vi "initialise.vi"(8 "error in (no error)":errorcluster, 11 "DL090201FrameScanTrajectory in":refnum<class "TrajectoryDL090201FrameScan.lvclass">) -> (0 "error out":errorcluster, 3 "DL090201FrameScanTrajectory out":refnum<class "TrajectoryDL090201FrameScan.lvclass">)   [LabVIEW 2010, in "TrajectoryDL090201FrameScan.lvclass"]
uses:
  TrajectoryDL090201FrameScan.lvclass
  TrajectoryDL091126GenericVoxel/TrajectoryDL091126GenericVoxel/TrajectoryDL091126GenericVoxel.lvclass
  common/enumerations/x_y_z_enumeration.ctl
  common/enumerations/functional_global_action_enum.ctl
  TrajectoryDL090201FrameScan.lvclass/TrajectoryDL090201FrameScan.ctl
  <vilib>/Analysis/1siggen.llb/Ramp Pattern by Samples.vi
  common/classes/ErrorController/ErrorController/class_data.vi
  common/classes/Box/Box/Box.lvclass
  common/classes/SpaceVector/SpaceVector/SpaceVector.lvclass
  <vilib>/Analysis/NI_AALBase.lvlib
  common/classes/ErrorController/ErrorController/ErrorController.lvclass
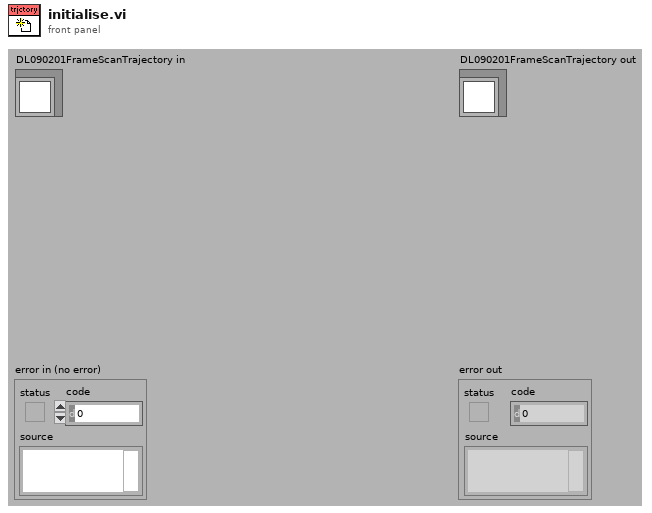
[diagram p1: front panel]
types:
  T1 = typedef "functional_global_action_enum.ctl" = enum16{"get", "set", "reset"}
  T2 = typedef "x_y_z_enumeration.ctl" = enum16{"x", "y", "z"}
  T3 = typedef "space_vector_array.ctl" = dbl[unit][]
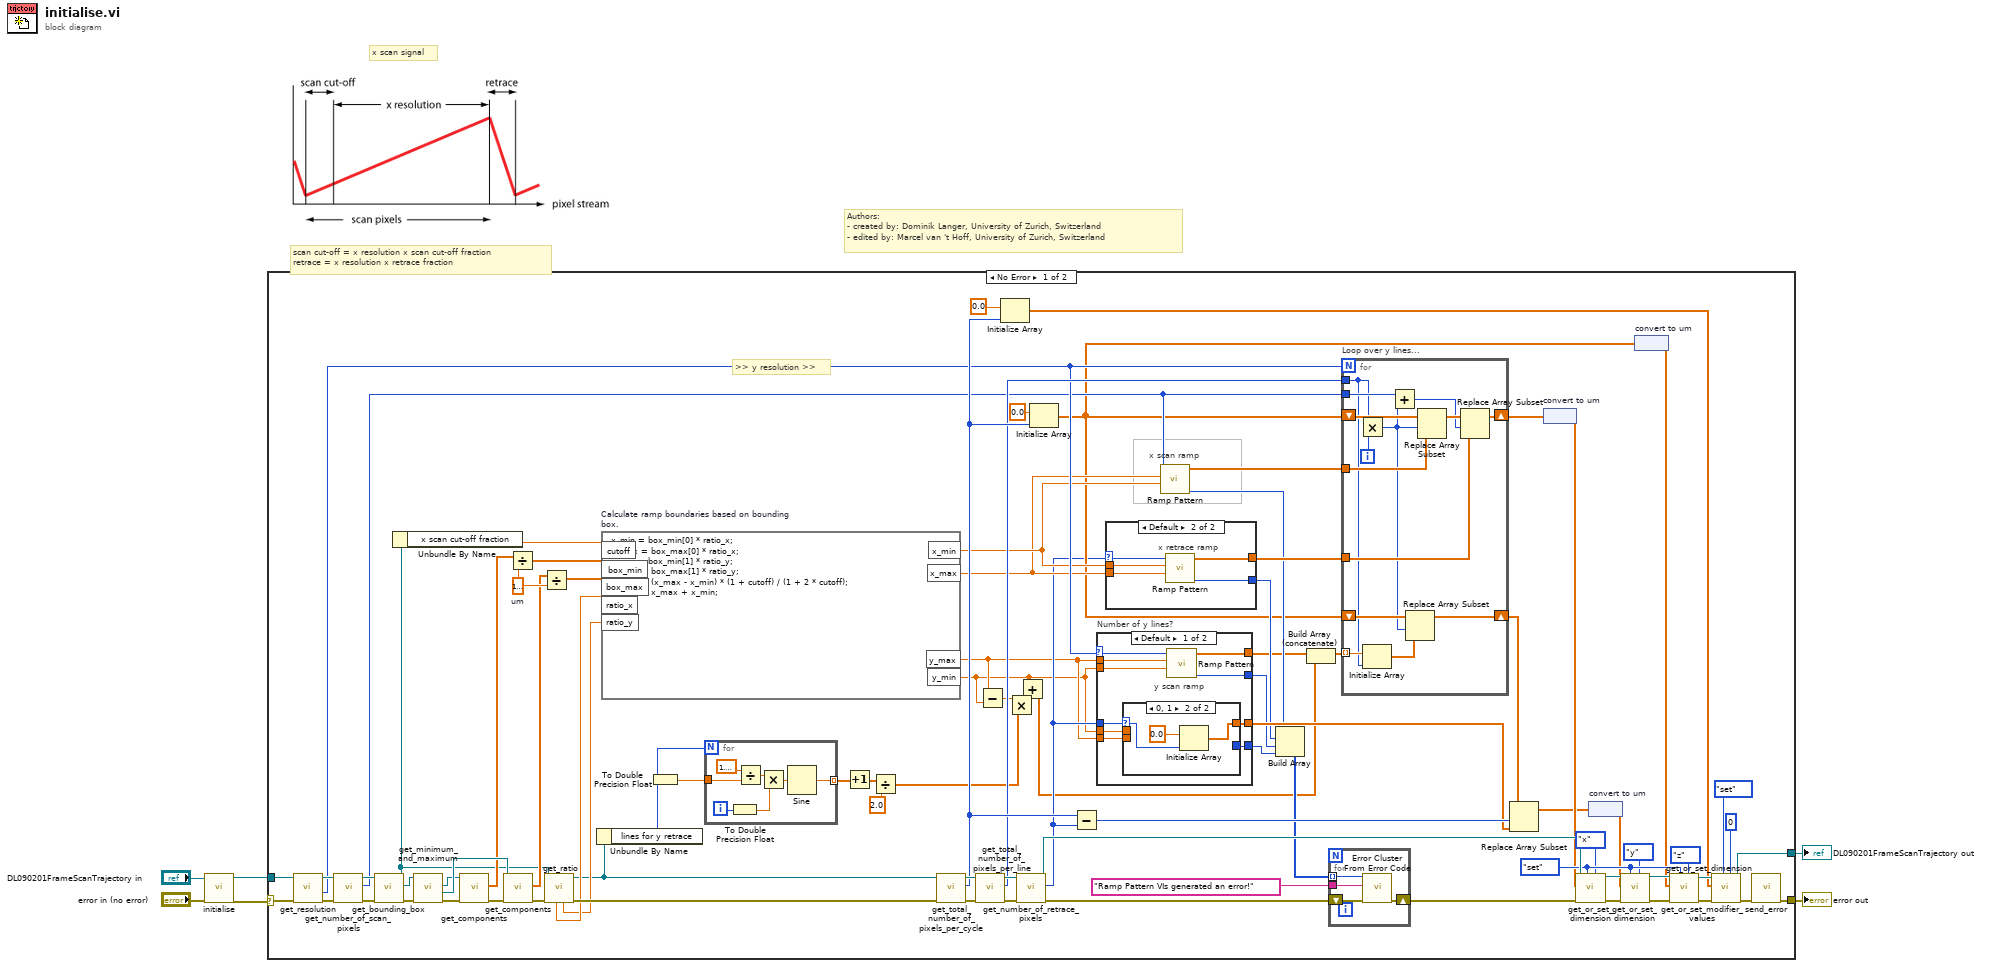
[diagram p0: block diagram]
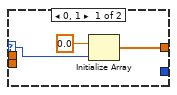
[diagram p2: hidden frame]
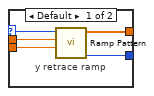
[diagram p3: hidden frame]
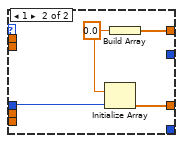
[diagram p4: hidden frame]
diagram:
  # "scan cut-off = x resolution x scan cut-off fraction\nretrace = x resolution x retrace fraction"
  # "x scan signal"
  # "Authors: \n- created by: Dominik Langer, University of Zurich, Switzerland\n- edited by: Marcel van 't Hoff, University of Zurich, Switzerland"
  n1 = call-parent "initialise.vi"("error in (no error)"="error in (no error)", "GenericTrajectory in"="DL090201FrameScanTrajectory in") -> ("error out"=w3:errorcluster, "GenericTrajectory out"=w1:refnum<class "TrajectoryDL090201FrameScan.lvclass">)  [unwired: 8 out]
  n2 = case shown="No Error" w3 {
    selector: w3 -> [w70 w149]
    tunnel: [w46 w149] -> w6
    tunnel: [w48 w148] -> w5
    tunnel: w1 -> [w29 w148]
    frame No Error {
      w61 = functional_global_action_enum."set" ("action")
      w86 = dbl[unit] 1e-06  # um
      # ">> y resolution >>"
      # "x scan ramp"
      n3 = call-dynamic "get_resolution.vi"("error in (no error)"=w70, "TrajectoryDL090201FrameScan in"=w29) -> ("error out"=w69:errorcluster, "y"=w57:i32, "TrajectoryDL090201FrameScan out"=w68:refnum<class "TrajectoryDL090201FrameScan.lvclass">)  [unwired: 7 out]
      n4 = call "get_number_of_scan_pixels.vi"("error in (no error)"=w69, "DL090201FrameScanTrajectory in"=w68) -> ("error out"=w73:errorcluster, "number of scan pixels"=w31:i32, "DL090201FrameScanTrajectory out"=w72:refnum<class "TrajectoryDL090201FrameScan.lvclass">)  [unwired: 7 out]
      n5 = call-dynamic "get_bounding_box.vi"("error in (no error)"=w73, "GenericTrajectory in"=w72) -> ("error out"=w77:errorcluster, "Box.lvclass"=w76:refnum<class "Box.lvclass">, "GenericTrajectory out"=w28:refnum<class "TrajectoryDL090201FrameScan.lvclass">)  [unwired: 7 in]
      n6 = Unbundle By Name(w28) -> ("x scan cut-off fraction"=w30:dbl)
      n7 = call "get_minimum_and_maximum.vi"("error in (no error)"=w77, "Box in"=w76) -> ("error out"=w75:errorcluster, "maximum"=w65:refnum<class "SpaceVector.lvclass">, "minimum"=w64:refnum<class "SpaceVector.lvclass">)  [unwired: 7 out]
      n8 = call "get_components.vi"("error in (no error)"=w75, "SpaceVector in"=w64) -> ("error out"=w74:errorcluster, "x/y/z"=w37:T3)  [unwired: 8 out]
      n9 = call "get_components.vi"("error in (no error)"=w74, "SpaceVector in"=w65) -> ("error out"=w55:errorcluster, "x/y/z"=w33:T3)  [unwired: 8 out]
      n10 = Divide(x=w37, y=w86) -> (x/y=w36:dbl[])
      n11 = Divide(x=w33, y=w86) -> (x/y=w32:dbl[])
      n12 = call-dynamic "get_ratio.vi"("error in (no error)"=w55, "TrajectoryDL090201FrameScan in"=w28) -> ("error out"=w54:errorcluster, "TrajectoryDL090201FrameScan out"=w19:refnum<class "TrajectoryDL090201FrameScan.lvclass">, "y normalised"=w38:dbl, "x normalised"=w39:dbl)  [unwired: 6 out]
      n13 = Unbundle By Name(w19) -> ("lines for y retrace"=w18:i32)
      n14 = formula code="x_min = box_min[0] * ratio_x;\nx_max = box_max[0] * ratio_x;\ny_min = box_min[1] * ratio_y;\ny_max = box_max[1] * ratio_y;\nx_max = (x_max - x_min) * (1 + cutoff) / (1 + 2 * cutoff);\nx_max = x_max + x_min;" "Calculate ramp boundaries based on bounding box."("box_min"=w36, "box_max"=w32, "ratio_x"=w39, "ratio_y"=w38, "cutoff"=w30) -> ("x_min"=w35:dbl, "x_max"=w34:dbl, "y_min"=w11:dbl, "y_max"=w20:dbl)
      n15 = To Double Precision Float(number=w18) -> (double precision float=w17:dbl)
      n16 = for {
        N: w18 -> [_]
        tunnel: [w99] -> w15 mode=indexing
        tunnel: w17 -> [w98]
        i -> [w96]
        n17 = To Double Precision Float(number=w96) -> (double precision float=w95:dbl)
        n18 = Divide(x=1.5707963267948966, y=w98) -> (x/y=w97:dbl)
        n19 = Multiply(x=w97, y=w95) -> (x*y=w94:dbl)
        n20 = Sine(x=w94) -> (sin(x)=w99:dbl)
      }
      n21 = Increment(x=w15) -> (x+1=w14:dbl[])
      n22 = Divide(x=w14, y=2.0) -> (x/y=w10:dbl[])
      n23 = call-dynamic "get_total_number_of_pixels_per_cycle.vi"("error in (no error)"=w54, "TrajectoryDL090201FrameScan in"=w19) -> ("error out"=w81:errorcluster, "total number of pixels per cycle"=w67:i32, "TrajectoryDL090201FrameScan out"=w79:refnum<class "TrajectoryDL090201FrameScan.lvclass">)  [unwired: 7 out]
      n24 = call-dynamic "get_total_number_of_pixels_per_line.vi"("error in (no error)"=w81, "DL090201FrameScanTrajectory in"=w79) -> ("error out"=w80:errorcluster, "total number of pixels per line"=w66:i32, "DL090201FrameScanTrajectory out"=w78:refnum<class "TrajectoryDL090201FrameScan.lvclass">)  [unwired: 7 out]
      n25 = Subtract(x=w20, y=w11) -> (x-y=w16:dbl)
      n26 = Initialize Array(0.0 ("element"), w67) -> (w50:dbl[])
      n27 = Multiply(x=w16, y=w10) -> (x*y=w12:dbl[])
      n28 = call "get_number_of_retrace_pixels.vi"("error in (no error)"=w80, "DL090201FrameScanTrajectory in"=w78) -> ("error out"=w62:errorcluster, "number of retrace pixels"=w21:i32, "DL090201FrameScanTrajectory out"=w63:refnum<class "TrajectoryDL090201FrameScan.lvclass">)  [unwired: 7 out]
      n29 = Add(x=w11, y=w12) -> (x+y=w7:dbl[])
      n30 = Initialize Array(0.0 ("element"), w67) -> (w25:dbl[])
      n31 = Subtract(x=w67, y=w21) -> (x-y=w89:i32)
      n32 = case "Number of y lines?" shown="Default" w57 {
        selector: w57 -> [w113 _]
        tunnel: [w121 w133] -> w8
        tunnel: w20 -> [w120 _]
        tunnel: w11 -> [w119 _]
        tunnel: [w118 _] -> w42
        tunnel: [w117 _] -> w40
        tunnel: [w116 w131] -> w56
        tunnel: w21 -> [w112 w130]
        tunnel: w11 -> [w115 _]
        tunnel: w20 -> [w114 _]
        frame Default {
          # "y scan ramp"
          n33 = case shown="0, 1" w112 {
            selector: w112 -> [w122 w129]
            tunnel: [w126 _] -> w117
            tunnel: [w125 w127] -> w116
            tunnel: w115 -> [w124 _]
            tunnel: w114 -> [w123 _]
            frame Default {
              # "y retrace ramp"
              n34 = call-poly <vilib>:"Ramp Pattern.vi"("start"=w123, "end"=w124, "samples"=w122) -> ("error"=w126:i32, "Ramp Pattern"=w125:dbl[])  [unwired: 7 in]
            }
            frame 0, 1 {
              n35 = Initialize Array(0.0 ("element"), w129) -> (w127:dbl[])
            }
          }
          n36 = call-poly <vilib>:"Ramp Pattern.vi"("start"=w119, "end"=w120, "samples"=w113) -> ("error"=w118:i32, "Ramp Pattern"=w121:dbl[])  [unwired: 7 in]
        }
        frame 1 {
          w132 = 0.0 ("element")
          n37 = Initialize Array(w132, w130) -> (w131:dbl[])
          n38 = Build Array(w132) -> (w133:dbl[])
        }
      }
      n39 = case shown="Default" w21 {
        selector: w21 -> [w101 w103]
        tunnel: [w100 w107] -> w90
        tunnel: [_ w106] -> w43
        tunnel: w35 -> [_ w105]
        tunnel: w34 -> [_ w104]
        frame 0, 1 {
          n40 = Initialize Array(0.0 ("element"), w101) -> (w100:dbl[])
        }
        frame Default {
          # "x retrace ramp"
          n41 = call-poly <vilib>:"Ramp Pattern.vi"("start"=w104, "end"=w105, "samples"=w103) -> ("error"=w106:i32, "Ramp Pattern"=w107:dbl[])  [unwired: 7 in]
        }
      }
      n42 = call-poly <vilib>:"Ramp Pattern.vi"("start"=w35, "end"=w34, "samples"=w31) -> ("error"=w44:i32, "Ramp Pattern"=w91:dbl[])  [unwired: 7 in]
      n43 = Build Array(w44, w43, w42, w40) -> (w41:i32[])
      n44 = Build Array (concatenate)(w8, w7) -> (w9:dbl[])
      n45 = for {
        tunnel: "Ramp Pattern VIs generated an error!" ("error message (\"\")") -> [w111]
        tunnel: w41 -> [w109] mode=indexing
        shift-right: [w108] -> w45
        shift-left: w62 -> [w110]
        n46 = call <vilib>:"Error Cluster From Error Code.vi"("error in (no error)"=w110, "error message (\"\")"=w111, "error code (0)"=w109) -> ("error out"=w108:errorcluster)  [unwired: 1 in, 5 out]
      }
      n47 = for "Loop over y lines..." {
        N: w57 -> [_]
        tunnel: w91 -> [w145]
        shift-right: [w146] -> w27
        shift-left: w25 -> [w147]
        tunnel: w90 -> [w144]
        tunnel: w9 -> [w141] mode=indexing
        shift-right: [w138] -> w88
        shift-left: w25 -> [w142]
        tunnel: w66 -> [w136]
        tunnel: w31 -> [w137]
        i -> [w143]
        n48 = Multiply(x=w136, y=w143) -> (x*y=w139:i32)
        n49 = Initialize Array(w141, w136) -> (w140:dbl[])
        n50 = Add(x=w137, y=w139) -> (x+y=w134:i32)
        n51 = Replace Array Subset(array=w142, new element=w140, index=w139) -> (w138:dbl[])
        n52 = Replace Array Subset(array=w147, new element=w145, index=w139) -> (w135:dbl[])
        n53 = Replace Array Subset(array=w135, new element=w144, index=w134) -> (w146:dbl[])
      }
      n54 = Replace Array Subset(array=w88, new element=w56, index=w89) -> (w23:dbl[])
      n55 = node "convert to um"(w27) -> (w26:dbl[unit][])
      n56 = call-dynamic "get_or_set_dimension.vi"("dimension"=x_y_z_enumeration."x", "action"=w61, "error in (no error)"=w45, "pixel values in (single dimension)"=w26, "GenericTrajectory in"=w63) -> ("error out"=w83:errorcluster, "GenericTrajectory out"=w85:refnum<class "TrajectoryDL090201FrameScan.lvclass">)  [unwired: 1 in, 4 out]
      n57 = node "convert to um"(w23) -> (w22:dbl[unit][])
      n58 = call-dynamic "get_or_set_dimension.vi"("dimension"=x_y_z_enumeration."y", "action"=w61, "error in (no error)"=w83, "pixel values in (single dimension)"=w22, "GenericTrajectory in"=w85) -> ("error out"=w82:errorcluster, "GenericTrajectory out"=w84:refnum<class "TrajectoryDL090201FrameScan.lvclass">)  [unwired: 1 in, 4 out]
      n59 = node "convert to um"(w25) -> (w24:dbl[unit][])
      n60 = call-dynamic "get_or_set_dimension.vi"("dimension"=x_y_z_enumeration."z", "action"=w61, "error in (no error)"=w82, "pixel values in (single dimension)"=w24, "GenericTrajectory in"=w84) -> ("error out"=w53:errorcluster, "GenericTrajectory out"=w52:refnum<class "TrajectoryDL090201FrameScan.lvclass">)  [unwired: 1 in, 4 out]
      n61 = call-dynamic "get_or_set_modifier_values.vi"("modifier index"=0, "action"=functional_global_action_enum."set", "error in (no error)"=w53, "modifier values in"=w50, "GenericTrajectory in"=w52) -> ("error out"=w47:errorcluster, "GenericTrajectory out"=w48:refnum<class "TrajectoryDL090201FrameScan.lvclass">)  [unwired: 4 in, 1 out]
      n62 = call "send_error.vi"("error in (no error)"=w47) -> ("error out"=w46:errorcluster)  [unwired: 10 in]
    }
    frame Error {
    }
  }
  "error out" <- w6
  "DL090201FrameScanTrajectory out" <- w5
